vi "Check_and_rewrite_file.vi"(0 "Filename":path, 7 "Present Channels only":bool, 9 "Present Channels":string[](array[string]), 11 "Start of read offset (chars.: 0)":i64) -> (4 "exists?":bool, 6 "Merged Channels":string[](array[string]), 8 "Start of data (bytes)":i64, 10 "No of bytes/row (approx)":i64, 14 "Current file size (bytes)":i64, 15 "Merged?":bool)   [LabVIEW 2022 SP3]
uses:
  <vilib>/Utility/error.llb/whitespace.ctl
  <vilib>/Utility/error.llb/Trim Whitespace One-Sided.vi
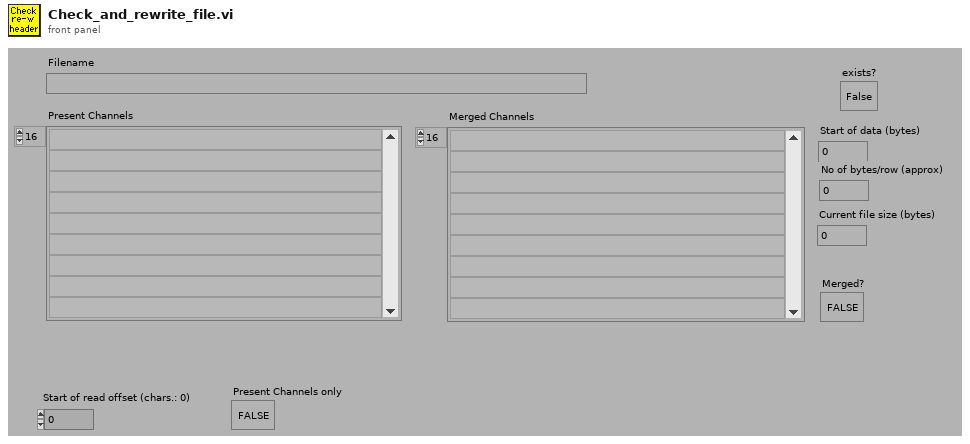
[diagram p1: front panel]
types:
  T1 = typedef "whitespace.ctl" = u16
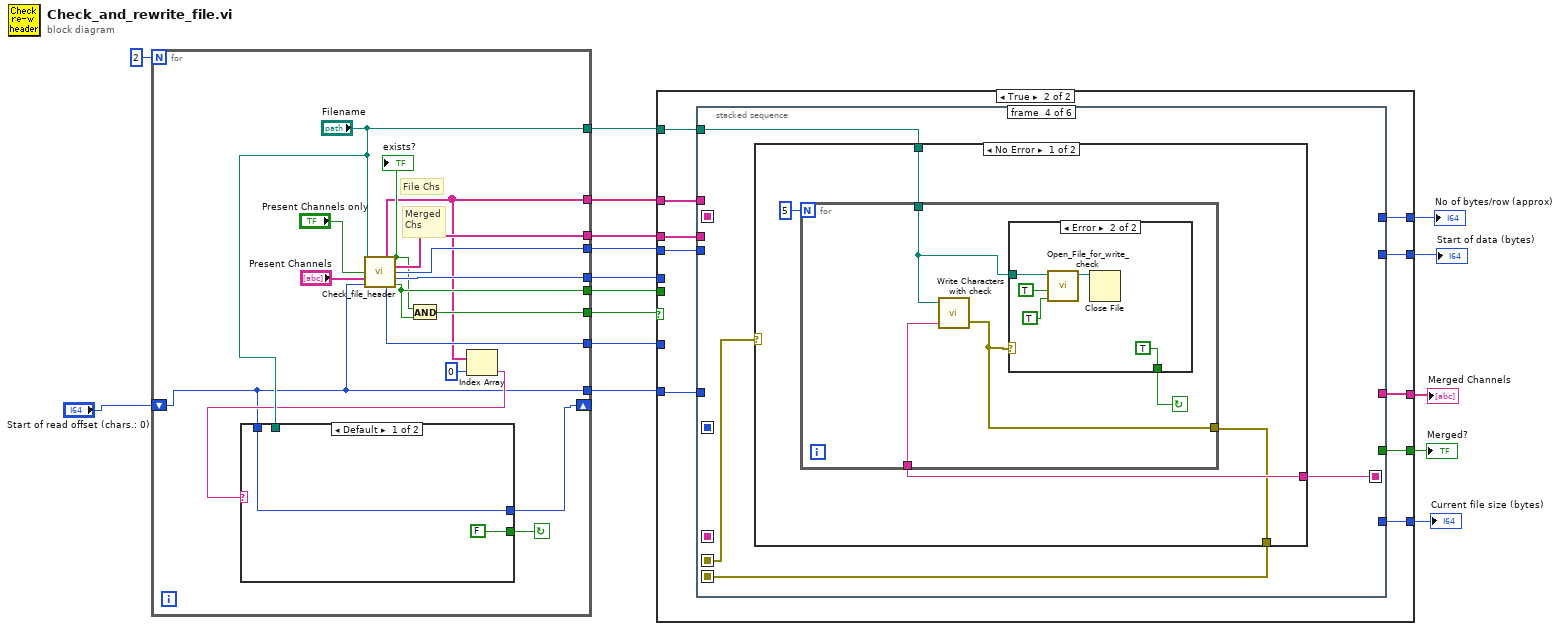
[diagram p0: block diagram]
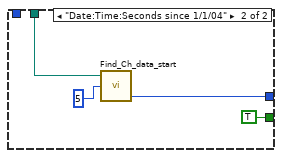
[diagram p2: hidden frame]
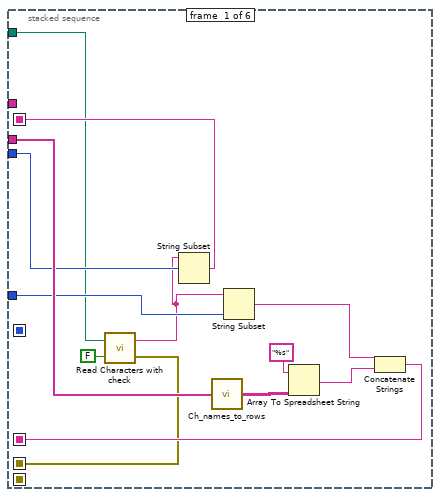
[diagram p4: hidden frame]
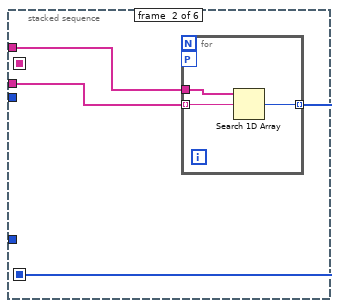
[diagram p5: hidden frame]
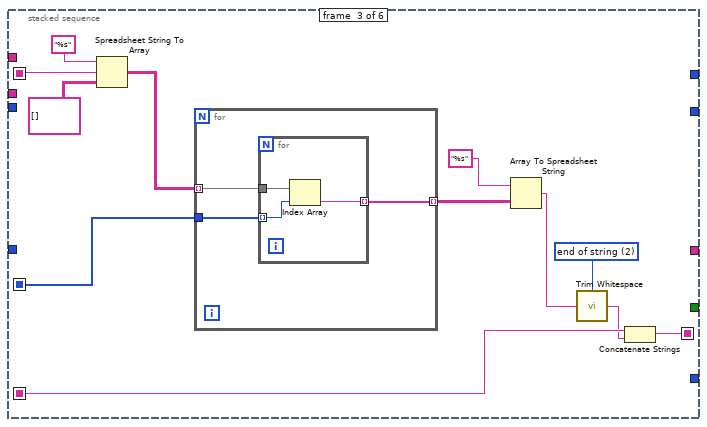
[diagram p6: hidden frame]
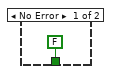
[diagram p7: hidden frame]
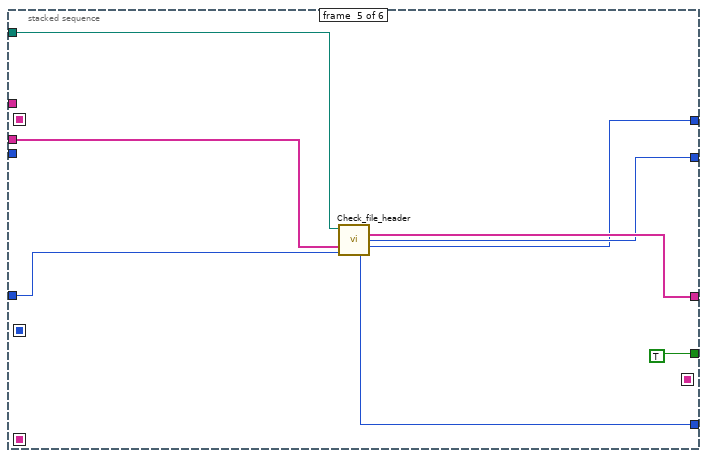
[diagram p9: hidden frame]
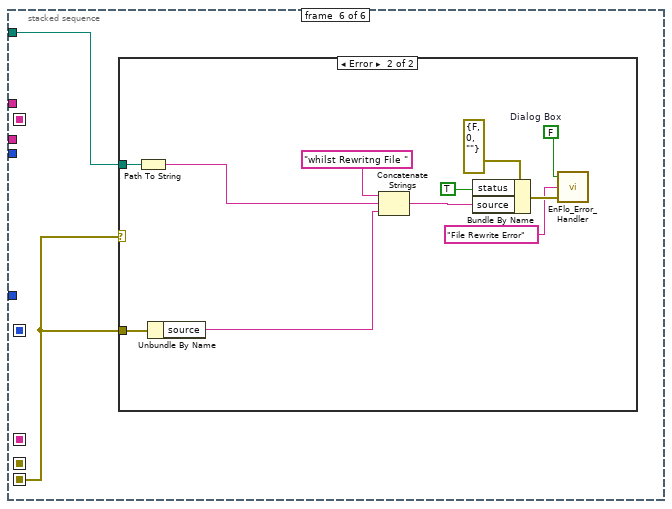
[diagram p10: hidden frame]
diagram:
  n1 = for {
    N: 2 -> [_]
    tunnel: [w32] -> w11
    tunnel: [w31] -> w10
    tunnel: [w30] -> w9
    tunnel: [w29] -> w8
    tunnel: [w28] -> w7
    tunnel: [w17] -> w6
    tunnel: [w22] -> w5
    tunnel: ["Filename"] -> w4
    tunnel: [w24] -> w3
    shift-right: [w19] -> _
    shift-left: "Start of read offset (chars.: 0)" -> [w17]
    stop <- w18 continue-if-true
    # "Merged\nChs"
    # "File Chs"
    n2 = call "Check_file_header.vi"("Filename"="Filename", "Present Channels only"="Present Channels only", "Present Channels"="Present Channels", "Start of read offset (chars.: 0)"=w17) -> ("File Channels"=w22:string[], "exists?"=w26:bool, "Merged Channels"=w31:string[], "Start of data (bytes)"=w30:i64, "No of bytes/row (approx)"=w29:i64, "Current file size (bytes)"=w28:i64, "Merged?"=w32:bool)  [unwired: 5 out]
    "exists?" <- w26
    n3 = And(x=w26, y=w32) -> (x .and. y?=w24:bool)
    n4 = Index Array(array=w22, index=0) -> (element=w20:string)
    n5 = case shown="Default" w20 {
      tunnel: "Filename" -> [_ w37]
      tunnel: [w33 w36] -> w19
      tunnel: [FALSE TRUE] -> w18
      tunnel: w17 -> [w33 _]
      frame Default {
      }
      frame "Date:Time:Seconds since 1/1/04" {
        n6 = call "Find_Ch_data_start.vi"("Approx No Of Columns"=5, "Filename"=w37) -> ("Start of read offset output"=w36:i32)  [unwired: 1 in, 2 out]
      }
    }
  }
  n7 = case shown="True" w3 {
    tunnel: [w42 w51] -> w16
    tunnel: [w43 w50] -> w15
    tunnel: [w40 w48] -> w14
    tunnel: [w41 w49] -> w13
    tunnel: [w39 w47] -> w12
    tunnel: w11 -> [w43 _]
    tunnel: w10 -> [w42 w52]
    tunnel: w9 -> [w41 w45]
    tunnel: w8 -> [w40 _]
    tunnel: w7 -> [w39 _]
    tunnel: w6 -> [_ w46]
    tunnel: w5 -> [_ w44]
    tunnel: w4 -> [_ w53]
    frame False {
    }
    frame True {
      n8 = stacked-sequence {
        seq-local: [_ w67 _ _ _ _] -> [_ _ w80 _ _ _]
        seq-local: [_ _ w76 _ _ _] -> [_ _ _ w94 _ _]
        seq-local: [w62 _ _ _ _ _] -> [_ _ w77 _ _ _]
        seq-local: [w58 _ _ _ _ _] -> [_ _ w84 _ _ _]
        seq-local: [w55 _ _ _ _ _] -> [_ _ _ w91 _ _]
        seq-local: [_ _ _ w92 _ _] -> [_ _ _ _ _ w118]
        tunnel: w53 -> [w57 _ _ w93 w116 w119]
        tunnel: w52 -> [w64 w69 _ _ w117 _]
        tunnel: [_ _ _ _ w115 _] -> w51
        tunnel: [_ _ _ _ TRUE _] -> w50
        tunnel: [_ _ _ _ w113 _] -> w49
        tunnel: [_ _ _ _ w112 _] -> w48
        tunnel: [_ _ _ _ w111 _] -> w47
        tunnel: w46 -> [w61 _ _ _ w110 _]
        tunnel: w45 -> [w59 _ _ _ _ _]
        tunnel: w44 -> [_ w68 _ _ _ _]
        frame #0 {
          n9 = call "Read Characters with check.vi"("Call EnFlo Error Handler?"=FALSE, "file (use dialog)"=w57) -> ("error out"=w55:errorcluster, "Read String"=w56:string)
          n10 = String Subset(string=w56, offset (0)=w59) -> (substring=w58:string)  [unwired: 1 in]
          n11 = call "Ch_names_to_rows.vi"("Channel Names"=w64) -> ("3 Row names"=w63:string[][])
          n12 = String Subset(string=w56, length (rest)=w61) -> (substring=w60:string)  [unwired: 1 in]
          n13 = Array To Spreadsheet String(array=w63, 3:"%s" ("format string")) -> (spreadsheet string=w65:string)  [unwired: 1 out]
          n14 = Concatenate Strings(w60, w65) -> (w62:string)
        }
        frame #1 {
          n15 = for {
            tunnel: w68 -> [w72]
            tunnel: w69 -> [w71] mode=indexing
            tunnel: [w70] -> w67 mode=indexing
            workers-P: _ -> [_]
            n16 = Search 1D Array(1D array=w72, element=w71) -> (index of element=w70:i32)  [unwired: 1 out]
          }
        }
        frame #2 {
          w73 = T1 2 items=["both", "start of string", "end of string"] ("location (both)")
          n17 = Spreadsheet String To Array(format string="%s", spreadsheet string=w84, array type (2D Dbl)=string[][] []) -> (array=w81:string[][])  [unwired: 1 in]
          n18 = for {
            tunnel: w81 -> [w87] mode=indexing
            tunnel: w80 -> [w86]
            tunnel: [w85] -> w79 mode=indexing
            n19 = for {
              tunnel: w87 -> [w90]
              tunnel: w86 -> [w89] mode=indexing
              tunnel: [w88] -> w85 mode=indexing
              n20 = Index Array(array=w90, index=w89) -> (element=w88:string)
            }
          }
          n21 = Array To Spreadsheet String(array=w79, 3:"%s") -> (spreadsheet string=w75:string)  [unwired: 1 in]
          n22 = call <vilib>:"Trim Whitespace.vi"("string"=w75, "location (both)"=w73) -> ("trimmed string"=w74:string)
          n23 = Concatenate Strings(w77, w74) -> (w76:string)
        }
        frame #3 {
          n24 = case shown="No Error" w91 {
            selector: w91 -> [_ w109]
            tunnel: w94 -> [w98 _]
            tunnel: w93 -> [w97 _]
            tunnel: [w96 w109] -> w92
            frame No Error {
              n25 = for {
                N: 5 -> [_]
                tunnel: w98 -> [w100]
                tunnel: w97 -> [w101]
                tunnel: [w99] -> w96
                stop <- w102 continue-if-true
                n26 = call "Write Characters with check.vi"("String to Write"=w100, "file (use dialog)"=w101) -> ("error out"=w99:errorcluster)  [unwired: 2 in]
                n27 = case shown="Error" w99 {
                  tunnel: w101 -> [_ w107]
                  tunnel: [FALSE TRUE] -> w102
                  frame No Error {
                  }
                  frame Error {
                    n28 = call "Open_File_for_write_check.vi"("advisory dialog? (display:T)"=TRUE, "append to file? (new file:F)"=TRUE, "file path"=w107) -> ("refnum"=w108:refnum<file>)  [unwired: 7 in, 1 out]
                    n29 = Close File(refnum=w108) -> ()  [unwired: 1 in, 2 out]
                  }
                }
              }
            }
            frame Error {
            }
          }
        }
        frame #4 {
          n30 = call "Check_file_header.vi"("Filename"=w116, "Present Channels"=w117, "Start of read offset (chars.: 0)"=w110) -> ("Merged Channels"=w115:string[], "Start of data (bytes)"=w113:i64, "No of bytes/row (approx)"=w112:i64, "Current file size (bytes)"=w111:i64)  [unwired: 1 in, 8 out]
        }
        frame #5 {
          n31 = case shown="Error" w118 {
            tunnel: w119 -> [_ w124]
            tunnel: w118 -> [_ w121]
            frame No Error {
            }
            frame Error {
              w127 = FALSE  # Dialog Box
              n32 = Path To String(path=w124) -> (string=w123:string)
              n33 = Unbundle By Name(w121) -> ("source"=w120:string)
              n34 = Concatenate Strings("whilst Rewritng File ", w123, w120) -> (w125:string)
              n35 = Bundle By Name(cluster=errorcluster {"status"=FALSE, "code"=0, "source"=""} ("error in (no error)"), "status"=TRUE ("Bundle Element"), "source"=w125) -> (w128:errorcluster)
              n36 = call "EnFlo_Error_Handler.vi"("error in (no error)"=w128, "Error Type"="File Rewrite Error", "Dialog Box (F)"=w127) -> ()  [unwired: 3 out]
            }
          }
        }
      }
    }
  }
  "Merged?" <- w15
  "Merged Channels" <- w16
  "Current file size (bytes)" <- w12
  "Start of data (bytes)" <- w13
  "No of bytes/row (approx)" <- w14
